vi "Drag.vi"(10 "offset":T1, 11 "Blob in":refnum<class "Blob.lvclass">) -> (3 "Blob out":refnum<class "Blob.lvclass">)   [LabVIEW 2019, in "Blob.lvclass"]
doc: "Move the bounds of the Blob to the specified offset."
uses:
  Blob.lvclass
  <vilib>/Utility/miscctls.llb/LVPoint32TypeDef.ctl
  Blob.lvclass/Blob.ctl
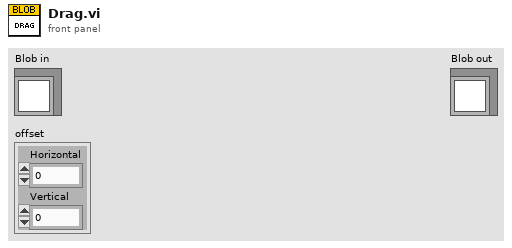
[diagram p1: front panel]
types:
  T1 = typedef "LVPoint32TypeDef.ctl" = cluster{"Horizontal":i32, "Vertical":i32}
  T2 = typedef "LVRectTypeDef.ctl" = cluster{"Left":i16, "Top":i16, "Right":i16, "Bottom":i16}
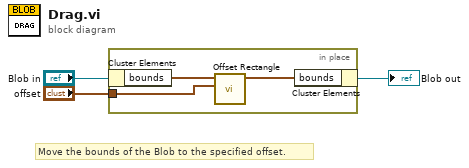
[diagram p0: block diagram]
diagram:
  # "Move the bounds of the Blob to the specified offset."
  n1 = in-place "In Place Element Structure" {
    in-place-border: "offset" -> [w4]
    n2 = in-place-cluster #1 ("Unbundle / Bundle Elements")("Blob in") -> ("bounds"=w6:T2)
    n3 = call "Offset Rectangle.vi"("offset"=w4, "rect in"=w6) -> ("rect out"=w5:T2)  [unwired: 9 in]
    n4 = in-place-cluster #1 ("Unbundle / Bundle Elements")("bounds"=w5) -> (→"Blob out":refnum<class "Blob.lvclass">)
  }
